vi "Update Data.vi"(8 "error in (no error)":errorcluster, 10 "Data":T1, 11 "Data Processor Module in":refnum<class "Data Processor Module.lvclass">) -> (0 "error out":errorcluster, 3 "Data Processor Module out":refnum<class "Data Processor Module.lvclass">)   [LabVIEW 2020, in "VolatusData.lvlib" / "Data Processor Module.lvclass"]
uses:
  Data Processor Module.lvclass
  C:/dev/lv20CE/relink/lv-volatus/Volatus/Module/Module.lvclass
  New Data.ctl
  Data Processor Module.lvclass/Data Processor Module.ctl
  lv-vecto/Vecto/Group DBL/Group DBL.lvclass
  C:/dev/lv20CE/relink/lv-vecto/Vecto/Group/Group.lvclass
  Volatus/Module/Module.lvclass/Module.ctl
  Volatus/VolatusAPI/VolatusAPI.lvclass/VolatusAPI.ctl
  <vilib>/Analysis/baseanly.llb/Mean (DBL).vi
  Volatus/Module/Module.lvclass
  <vilib>/Analysis/NI_AALBase.lvlib
  C:/dev/lv20CE/relink/lv-vecto/Vecto/Group DBL/Group DBL.lvclass
  C:/dev/lv20CE/relink/lv-volatus/VolatusData/Data Processor Module/Data Processor Module.lvclass
  VolatusData.lvlib
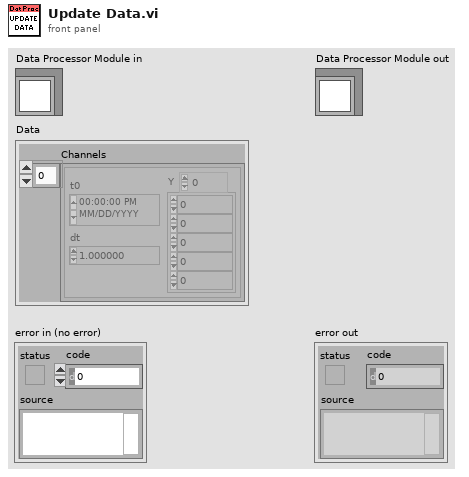
[diagram p1: front panel]
types:
  T1 = typedef "VolatusData.lvlib/New Data.ctl" = cluster{"Channels":waveform(dbl)[]}
  T2 = typedef "VolatusData.lvlib/Data Processor Module.lvclass/Decimation Type.ctl" = enum16{"Average", "Latest"}
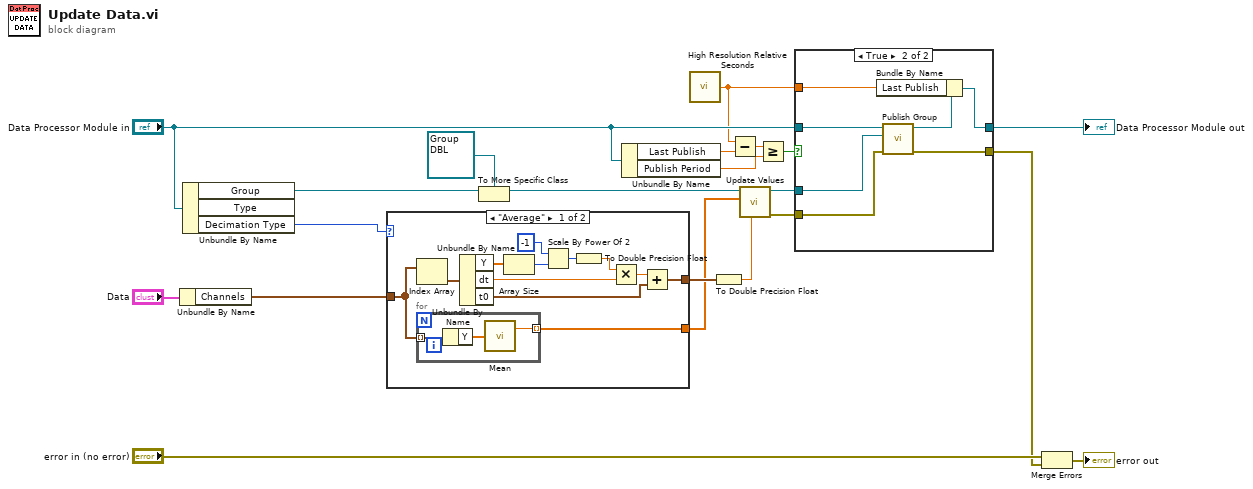
[diagram p0: block diagram]
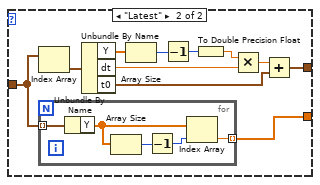
[diagram p2: hidden frame]
diagram:
  n1 = Unbundle By Name("Data") -> ("Channels"=w17:waveform(dbl)[])
  n2 = Unbundle By Name("Data Processor Module in") -> ("Group"=w16:refnum<class "Group.lvclass">, "Decimation Type"=w18:T2)  [unwired: 1 out]
  n3 = case shown="\"Average\"" w18 {
    tunnel: w17 -> [w23 w37]
    tunnel: [w24 w41] -> w15
    tunnel: [w22 w38] -> w13
    frame "Average" {
      n4 = Index Array(array=w23) -> (element=w29:waveform(dbl))  [unwired: 1 in]
      n5 = for {
        tunnel: [w34] -> w22 mode=indexing
        tunnel: w23 -> [w36] mode=indexing
        n6 = Unbundle By Name(w36) -> ("Y"=w35:dbl[])
        n7 = call-poly <vilib>:"Mean.vi"("X"=w35) -> ("mean"=w34:dbl)  [unwired: 1 out]
      }
      n8 = Unbundle By Name(w29) -> ("Y"=w30:dbl[], "dt"=w28:dbl, "t0"=w25:timestamp)
      n9 = Array Size(array=w30) -> (size(s)=w33:i32)
      n10 = Scale By Power Of 2(n=i16 -1, x=w33) -> (x*2^n=w31:i32)
      n11 = To Double Precision Float(number=w31) -> (double precision float=w27:dbl)
      n12 = Multiply(x=w27, y=w28) -> (x*y=w26:dbl)
      n13 = Add(x=w26, y=w25) -> (x+y=w24:timestamp)
    }
    frame "Latest" {
      n14 = Index Array(array=w37) -> (element=w46:waveform(dbl))  [unwired: 1 in]
      n15 = for {
        tunnel: [w51] -> w38 mode=indexing
        tunnel: w37 -> [w50] mode=indexing
        n16 = Unbundle By Name(w50) -> ("Y"=w49:dbl[])
        n17 = Array Size(array=w49) -> (size(s)=w52:i32)
        n18 = Decrement(x=w52) -> (x-1=w48:i32)
        n19 = Index Array(array=w49, index=w48) -> (element=w51:dbl)
      }
      n20 = Unbundle By Name(w46) -> ("Y"=w47:dbl[], "dt"=w45:dbl, "t0"=w42:timestamp)
      n21 = Array Size(array=w47) -> (size(s)=w40:i32)
      n22 = Decrement(x=w40) -> (x-1=w39:i32)
      n23 = To Double Precision Float(number=w39) -> (double precision float=w44:dbl)
      n24 = Multiply(x=w44, y=w45) -> (x*y=w43:dbl)
      n25 = Add(x=w43, y=w42) -> (x+y=w41:timestamp)
    }
  }
  n26 = To More Specific Class(target class=refnum<class "Group DBL.lvclass"> refnum ("Vecto.lvlib:Group DBL.lvclass"), reference=w16) -> (specific class reference=w7:refnum<class "Group DBL.lvclass">)  [unwired: 1 in, 1 out]
  n27 = Unbundle By Name("Data Processor Module in") -> ("Last Publish"=w5:dbl, "Publish Period"=w3:dbl)
  n28 = call <vilib>:"High Resolution Relative Seconds.vi"() -> ("relative seconds"=w1:dbl)
  n29 = To Double Precision Float(number=w15) -> (double precision float=w14:dbl)
  n30 = Subtract(x=w1, y=w5) -> (x-y=w4:dbl)
  n31 = call "Update Values.vi"("Timestamp (Now)"=w14, "Values"=w13, "Group in"=w7) -> ("error out"=w10:errorcluster, "Group out"=w11:refnum<class "Group DBL.lvclass">)  [unwired: 7 in]
  n32 = Greater Or Equal?(x=w4, y=w3) -> (x >= y?=w2:bool)
  n33 = case shown="True" w2 {
    tunnel: [w54 w56] -> w12
    tunnel: w11 -> [_ w60]
    tunnel: w10 -> [w53 w59]
    tunnel: [w53 w58] -> w8
    tunnel: "Data Processor Module in" -> [w54 w57]
    tunnel: w1 -> [_ w55]
    frame False {
    }
    frame True {
      n34 = call "Publish Group.vi"("error in (no error)"=w59, "Group"=w60, "Module in"=w57) -> ("error out"=w58:errorcluster, "Module out"=w61:refnum<class "Data Processor Module.lvclass">)  [unwired: 7 in]
      n35 = Bundle By Name(cluster=w61, "Last Publish"=w55) -> (w56:refnum<class "Data Processor Module.lvclass">)
    }
  }
  "Data Processor Module out" <- w12
  n36 = Merge Errors("error in (no error)", w8) -> (→"error out":errorcluster)
